vi "rad_Get Target Info.vi"(8 "error in (no error)":errorcluster, 11 "System Session in":refnum<k21>) -> (0 "error out":errorcluster, 2 "Target settings":T1={"Hostname"="", "Serial number"="", "Product name"="", "Product code"=0, "System status"="", "Credential type"=enum."None/Unlocked", "User added?"=FALSE, "Primary NIC"={"MAC address"="", "IP Address Request Mode"=2, "IP address"="", "Subnet mask"="", "Gateway"="", "DNS server"=""}} {"Primary NIC"."IP Address Request Mode" items=["Static"=1, "DHCP/Link-Local"=2, "Link-Local Only"=4, "DHCP Only"=8]}, 3 "System Session out":refnum<k21>)   [LabVIEW 2023]
uses:
  TypeDefs/rad_Target Information.ctl
  TypeDefs/rad_Target Network Settings.ctl
  <resource>/objmgr/nisysapi.rc
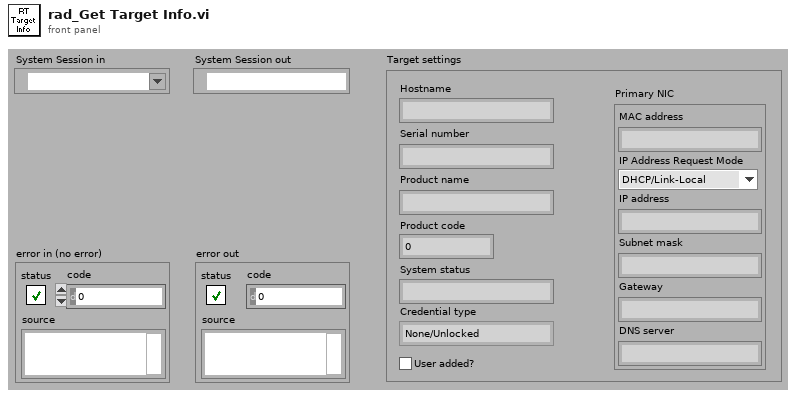
[diagram p1: front panel]
types:
  T1 = typedef "rad_Target Information.ctl" = cluster{"Hostname":string, "Serial number":string, "Product name":string, "Product code":i32, "System status":string, "Credential type":enum16{"None/Unlocked", "FTP Password", "NIAuth Credentials"}, "User added?":bool, "Primary NIC":T2}
  T2 = typedef "rad_Target Network Settings.ctl" = cluster{"MAC address":string, "IP Address Request Mode":i32, "IP address":string, "Subnet mask":string, "Gateway":string, "DNS server":string}
  T3 = enum16{"None/Unlocked", "FTP Password", "NIAuth Credentials"}
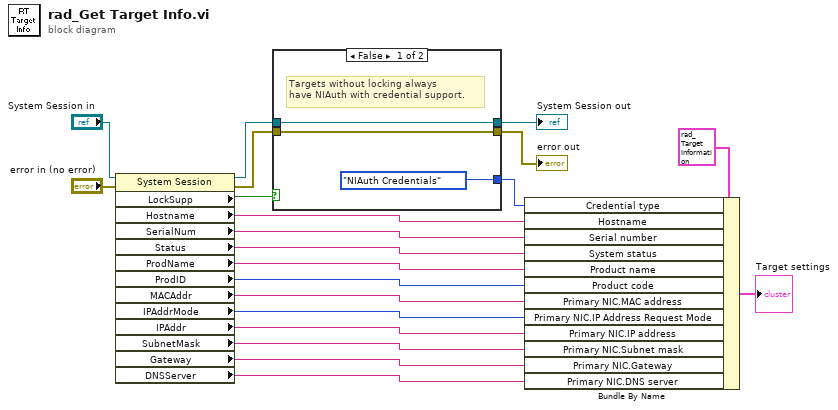
[diagram p0: block diagram]
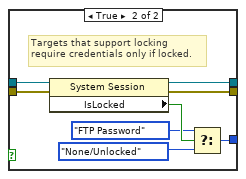
[diagram p2: hidden frame]
diagram:
  n1 = property class="System Session"(reference="System Session in", error in="error in (no error)") -> (reference out=w10:refnum<k21>, error out=w9:errorcluster, "LockSupp"=w8:bool, "Hostname"=w19:string, "SerialNum"=w17:string, "Status"=w16:string, "ProdName"=w15:string, "ProdID"=w14:i32, "MACAddr"=w13:string, "IPAddrMode"=w12:i32, "IPAddr"=w4:string, "SubnetMask"=w3:string, "Gateway"=w2:string, "DNSServer"=w1:string)
  n2 = case shown="False" w8 {
    tunnel: w10 -> [w24 w32]
    tunnel: w9 -> [w23 w31]
    tunnel: [w24 w30] -> w7
    tunnel: [w23 w29] -> w6
    tunnel: [T3."NIAuth Credentials" ("Credential type") w28] -> w5
    frame False {
      # "Targets without locking always\nhave NIAuth with credential support."
    }
    frame True {
      # "Targets that support locking\nrequire credentials only if locked."
      n3 = property class="System Session"(reference=w32, error in=w31) -> (reference out=w30:refnum<k21>, error out=w29:errorcluster, "IsLocked"=w27:bool)
      n4 = Select(t=T3."FTP Password" ("Credential type"), s=w27, f=T3."None/Unlocked" ("Credential type")) -> (s? t:f=w28:T3)
    }
  }
  "System Session out" <- w7
  "error out" <- w6
  n5 = Bundle By Name(cluster=T1 {"Hostname"="", "Serial number"="", "Product name"="", "Product code"=0, "System status"="", "Credential type"=enum."None/Unlocked", "User added?"=FALSE, "Primary NIC"={"MAC address"="", "IP Address Request Mode"=0, "IP address"="", "Subnet mask"="", "Gateway"="", "DNS server"=""}} ("Target settings"), "Credential type"=w5, "Hostname"=w19, "Serial number"=w17, "System status"=w16, "Product name"=w15, "Product code"=w14, "Primary NIC.MAC address"=w13, "Primary NIC.IP Address Request Mode"=w12, "Primary NIC.IP address"=w4, "Primary NIC.Subnet mask"=w3, "Primary NIC.Gateway"=w2, "Primary NIC.DNS server"=w1) -> (→"Target settings":T1)
